vi "SCL_for_R_W_I2C.vi"   [LabVIEW 2019]
uses:
  <vilib>/rvi/Emulation/niFpgaGetClockAttributes.vi
  <vilib>/rvi/Emulation/niFpgaSctlEmulationGetInTimedLoop.vi
  <vilib>/rvi/Emulation/niFpgaEmulationReportErrorSimple.vi
  <vilib>/rvi/eio/common/nirviEmuTemplateMethod_errors.vi
  <vilib>/rvi/Emulation/niFpgaCriticalErrorInLSC.vi
  <vilib>/eio/EIONode/EIONode.xnode
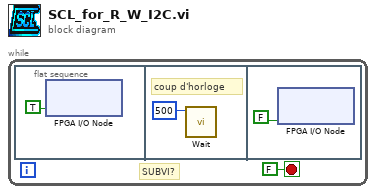
[diagram p0: block diagram]
diagram:
  n1 = while {
    stop <- FALSE stop-if-true
    # "SUBVI?"
    n2 = flat-sequence {
      frame #0 {
        n3 = xnode "FPGA I/O Node"("CLK"=TRUE) -> ()  [unwired: 1 in, 1 out]
      }
      frame #1 {
        # "coup d'horloge"
        n4 = call "Wait"("Count(Ticks)"=u32 500) -> ()  [unwired: 1 out]
      }
      frame #2 {
        n5 = xnode "FPGA I/O Node"("CLK"=FALSE) -> ()  [unwired: 1 in, 1 out]
      }
    }
  }
